vi "FindWedgeh.vi"(0 "Case Number":i32, 1 "cap theta":dbl[](array[numeric]) format="%.2f", 2 "rmin out":dbl format="%.2f", 3 "Sigma":dbl[](array[numeric]) format="%.2f", 4 "slice thetas":dbl[][](array[numeric]) format="%.4f", 5 "slice delay points in":i32, 6 "r values":T1 {"r5" format="%.2f"; "r4" format="%.2f"; "r3" format="%.2f"; "r2" format="%.2f"; "r1" format="%.2f"; "r0" format="%.2f"}, 7 "P constants":T3 {"Dtemp" format="%.2f"; "B" format="%.2f"; "A" format="%.2f"; "thetaw" format="%.2f"; "phih" format="%.2f"; "r" format="%.2f"}, 8 "strip":cluster{"Radius":dbl, "h":dbl, "a":dbl}={"Radius"=10.0, "h"=3.0, "a"=5.0} {"Radius" format="%.2f"; "a" format="%.2f"; "h" format="%.2f"}, 9 "P":cluster{"x":dbl, "y":dbl, "z":dbl}={"x"=1.0, "y"=-5.0, "z"=2.0} {"x" format="%.2f"; "z" format="%.2f"; "y" format="%.2f"}, 10 "Variables":T2={"sound spd (cm/s)"=150000, "time step (s)"=1e-09} {"time step (s)" format="%.2e"}, 11 "Transform matrix":dbl[][](array[numeric]) format="%.2f") -> (16 "h wedge":dbl[](graph), 18 "slice delay out":i32)   [LabVIEW 2022 SP3]
uses:
  <vilib>/Analysis/baseanly.llb/A x Vector.vi
  <vilib>/Analysis/NI_AALBase.lvlib
panel:
  out "x/y temp":T1 {"r5" format="%.2f"; "r4" format="%.2f"; "r3" format="%.2f"; "r2" format="%.2f"; "r1" format="%.2f"; "r0" format="%.2f"}
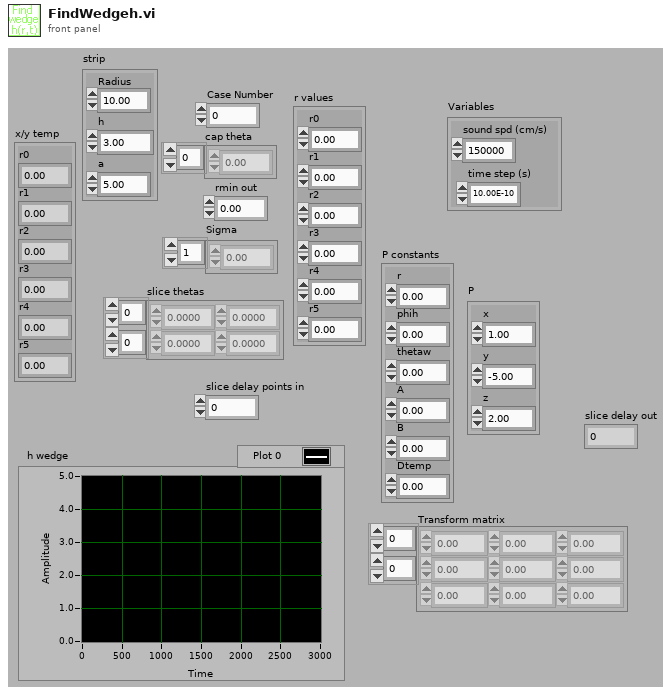
[diagram p1: front panel]
types:
  T1 = cluster{"r0":dbl, "r1":dbl, "r2":dbl, "r3":dbl, "r4":dbl, "r5":dbl}
  T2 = cluster{"sound spd (cm/s)":i32, "time step (s)":sgl}
  T3 = cluster{"r":dbl, "phih":dbl, "thetaw":dbl, "A":dbl, "B":dbl, "Dtemp":dbl}
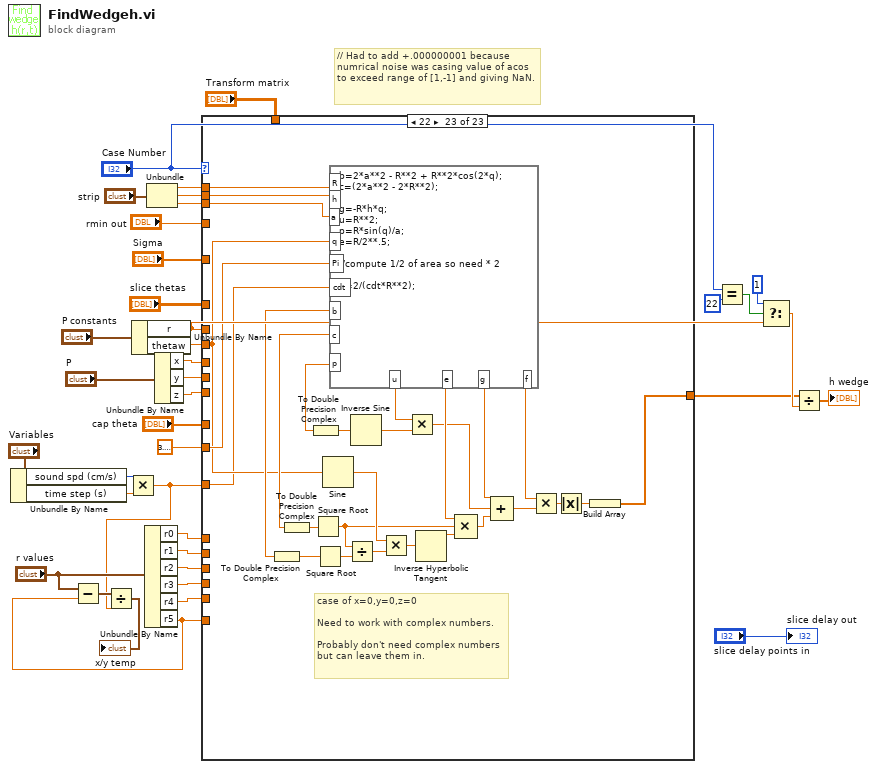
[diagram p0: block diagram]
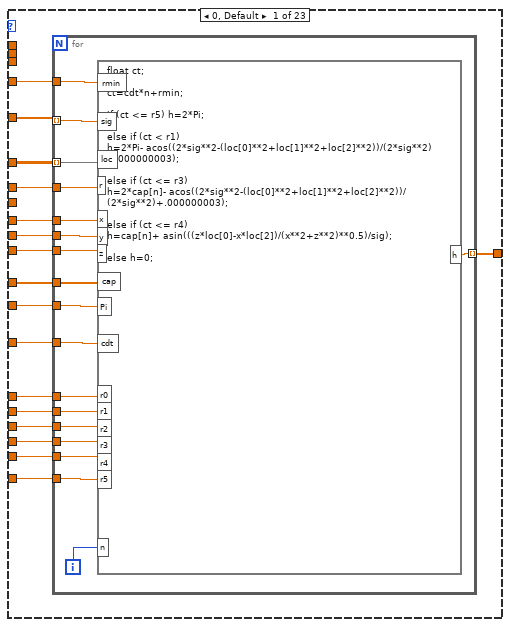
[diagram p2: hidden frame]
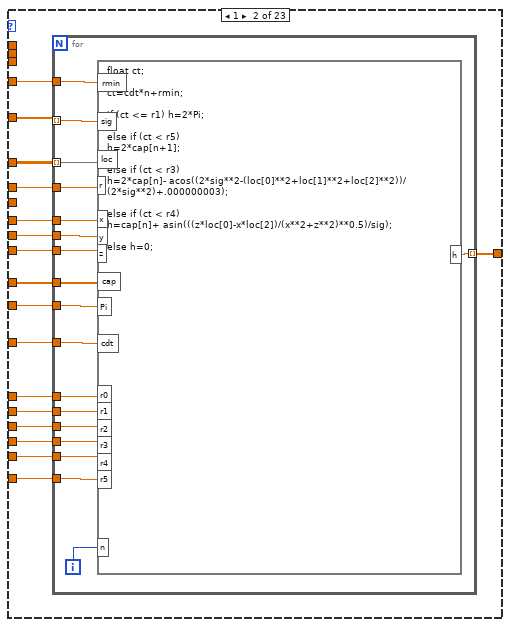
[diagram p3: hidden frame]
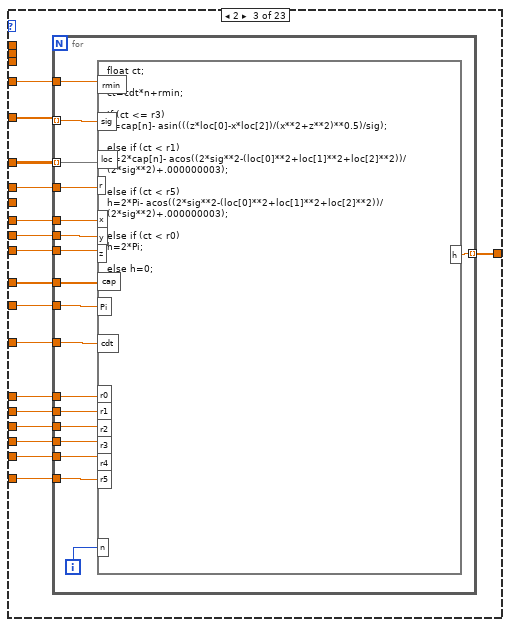
[diagram p4: hidden frame]
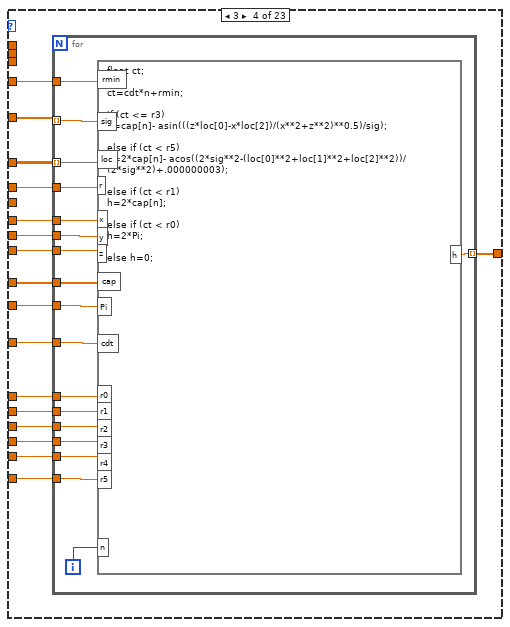
[diagram p5: hidden frame]
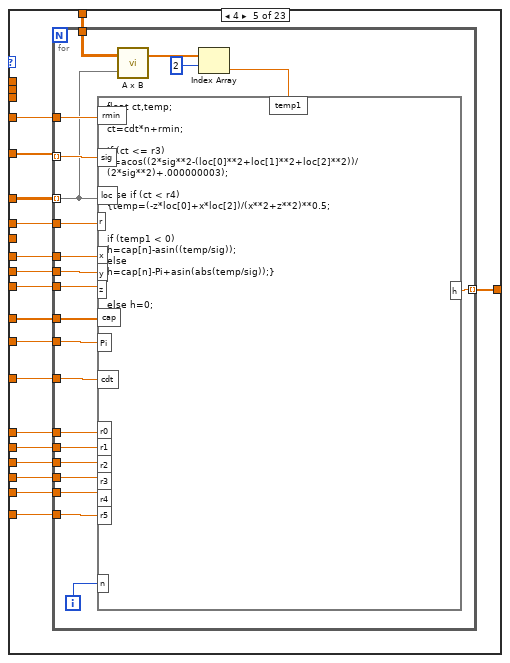
[diagram p6: hidden frame]
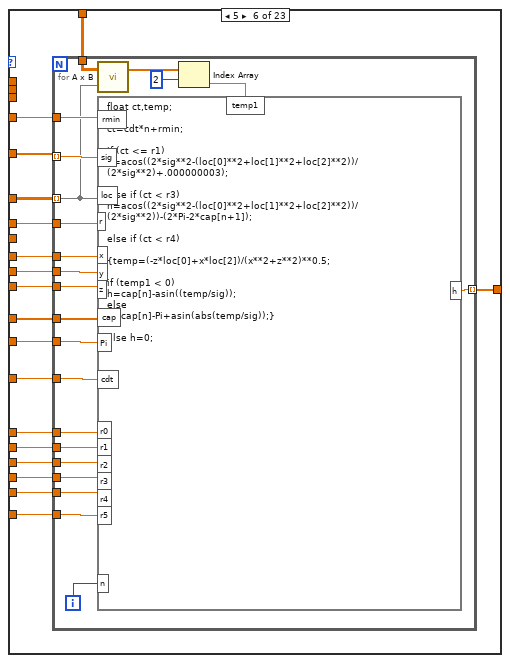
[diagram p7: hidden frame]
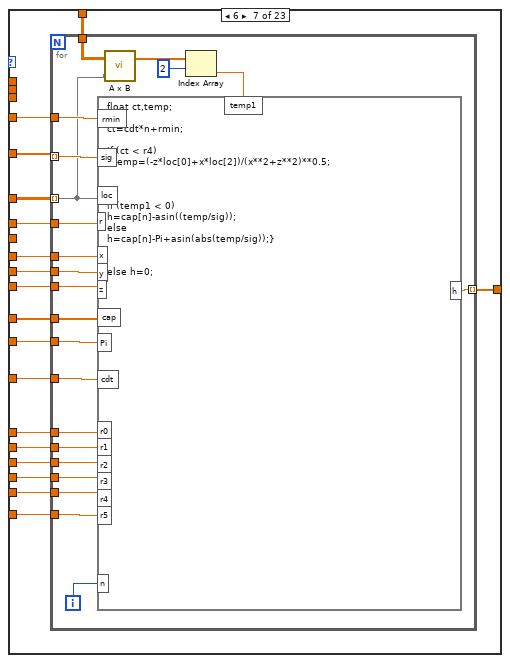
[diagram p8: hidden frame]
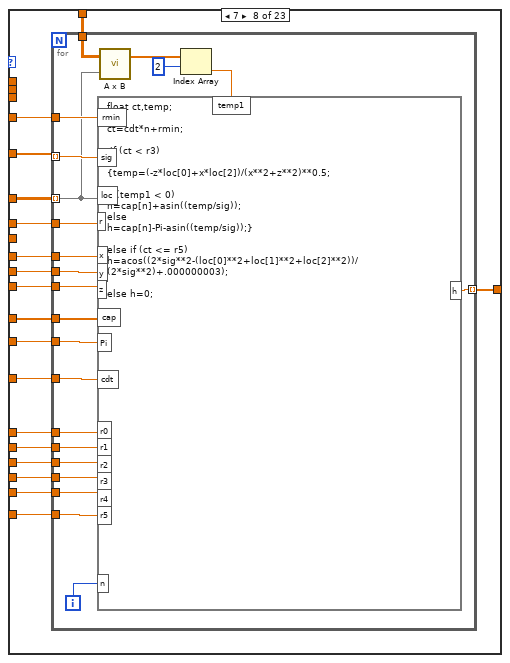
[diagram p9: hidden frame]
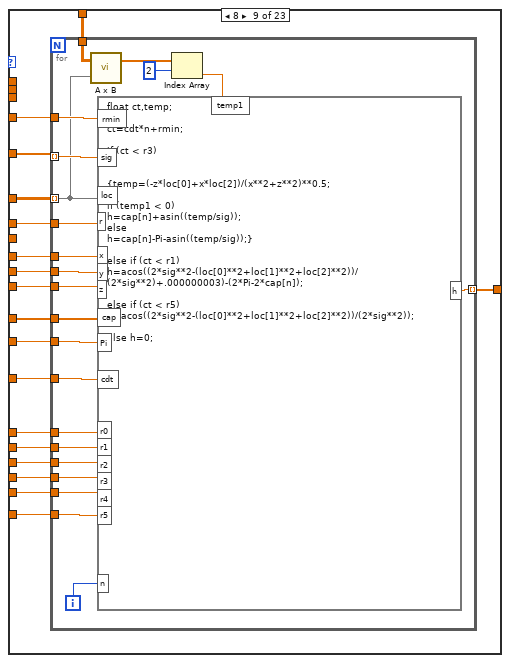
[diagram p10: hidden frame]
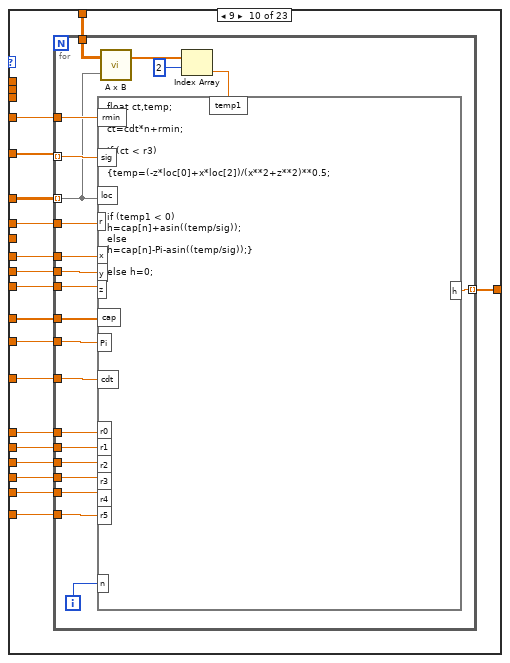
[diagram p11: hidden frame]
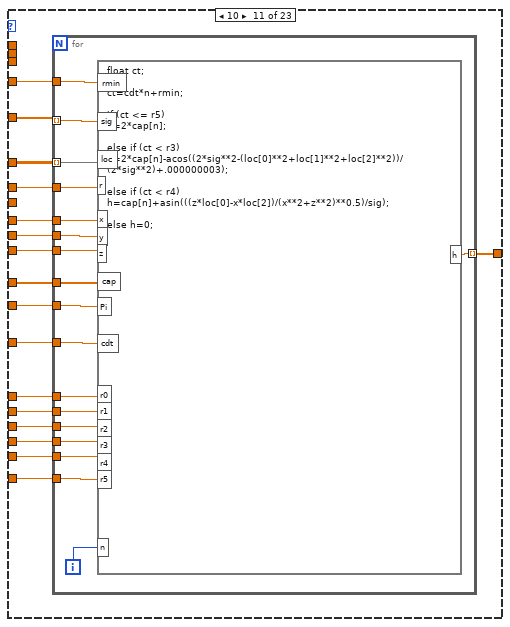
[diagram p12: hidden frame]
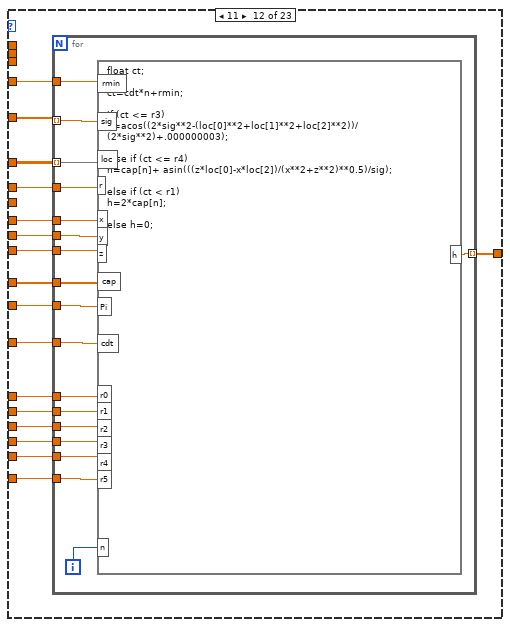
[diagram p13: hidden frame]
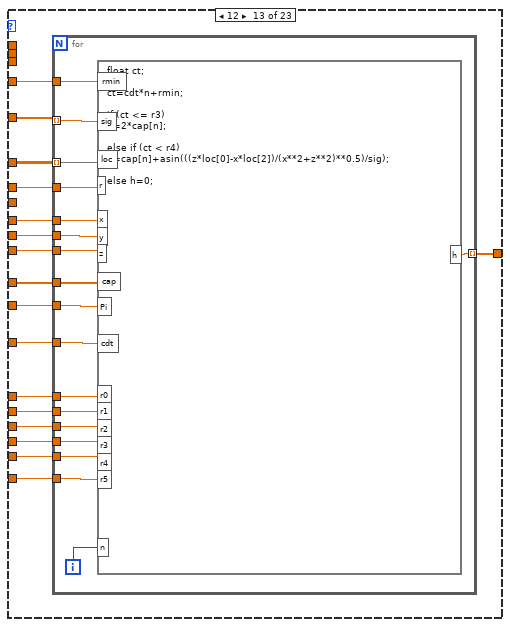
[diagram p14: hidden frame]
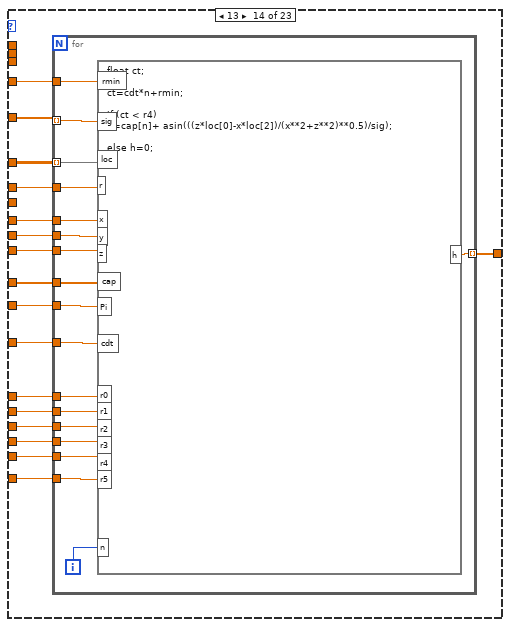
[diagram p15: hidden frame]
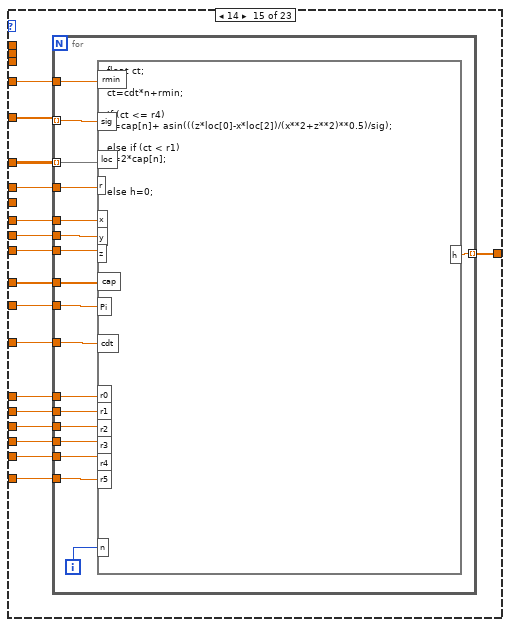
[diagram p16: hidden frame]
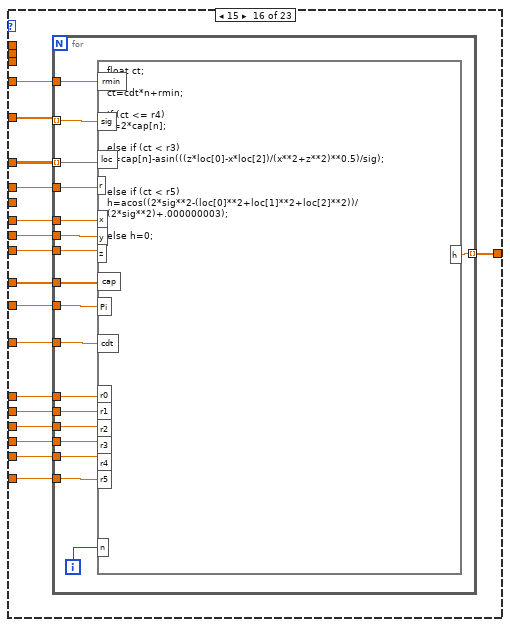
[diagram p17: hidden frame]
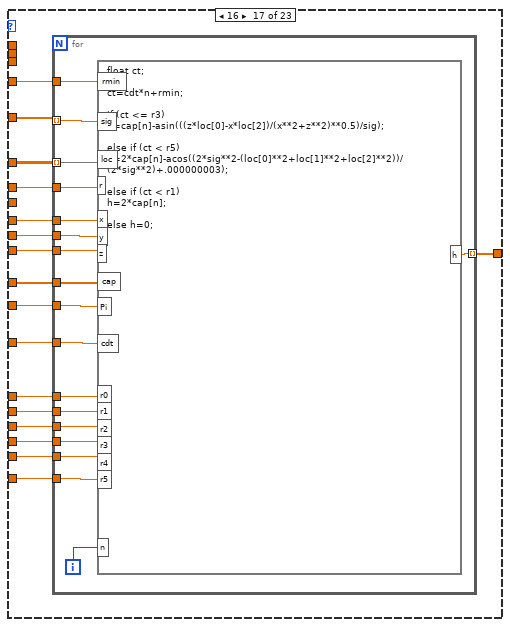
[diagram p18: hidden frame]
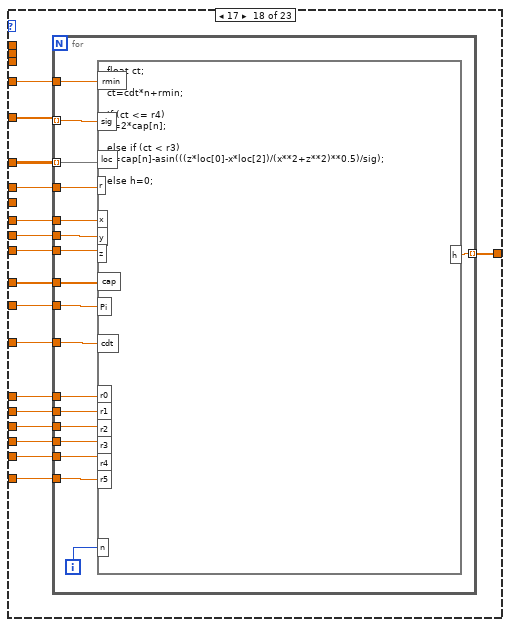
[diagram p19: hidden frame]
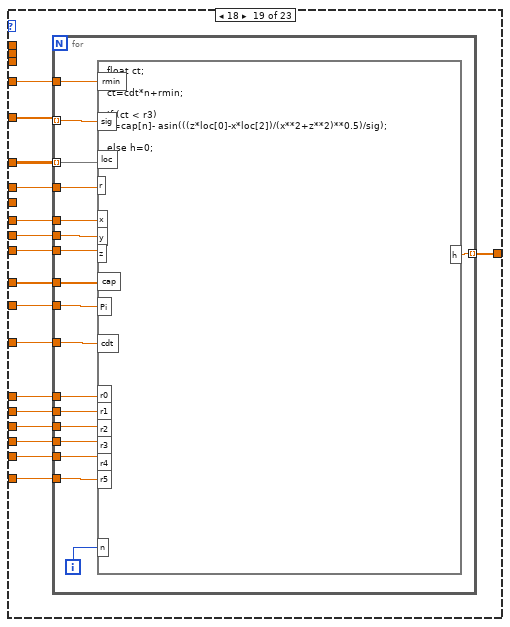
[diagram p20: hidden frame]
diagram:
  # "// Had to add +.000000001 because numrical noise was casing value of acos to exceed range of [1,-1] and giving NaN."
  n1 = Unbundle By Name("Variables") -> ("sound spd (cm/s)"=w26:i32, "time step (s)"=w7:sgl)
  n2 = Multiply(x=w26, y=w7) -> (x*y=w25:sgl)
  n3 = Unbundle By Name("P constants") -> ("r"=w8:dbl, "thetaw"=w18:dbl)
  n4 = Unbundle By Name("r values") -> ("r0"=w27:dbl, "r1"=w20:dbl, "r2"=w22:dbl, "r3"=w21:dbl, "r4"=w5:dbl, "r5"=w4:dbl)
  n5 = Subtract(x="r values", y=w4) -> (x-y=w30:T1)
  n6 = Divide(x=w30, y=w25) -> (x/y=→"x/y temp":T1)
  n7 = Unbundle("strip") -> ("Radius"=w10:dbl, "h"=w16:dbl, "a"=w15:dbl)
  n8 = Unbundle By Name("P") -> ("x"=w34:dbl, "y"=w33:dbl, "z"=w32:dbl)
  n9 = case shown="22" "Case Number" {
    tunnel: "cap theta" -> [w54 w89 w124 w159 w195 w235 w275 w315 w355 w395 w434 w469 w504 w539 w574 w609 w644 w679 w714 w749 w784 w819 _]
    tunnel: w25 -> [w55 w90 w125 w160 w196 w236 w276 w316 w356 w396 w435 w470 w505 w540 w575 w610 w645 w680 w715 w750 w785 w820 w846]
    tunnel: "slice thetas" -> [w41 w76 w111 w146 w182 w222 w262 w302 w342 w382 w421 w456 w491 w526 w561 w596 w631 w666 w701 w736 w771 w806 _]
    tunnel: w8 -> [w53 w88 w123 w158 w194 w234 w274 w314 w354 w394 w433 w468 w503 w538 w573 w608 w643 w678 w713 w748 w783 w818 _]
    tunnel: w27 -> [w52 w87 w122 w157 w193 w233 w273 w313 w353 w393 w432 w467 w502 w537 w572 w607 w642 w677 w712 w747 w782 w817 _]
    tunnel: w20 -> [w51 w86 w121 w156 w192 w232 w272 w312 w352 w392 w431 w466 w501 w536 w571 w606 w641 w676 w711 w746 w781 w816 _]
    tunnel: w22 -> [w50 w85 w120 w155 w191 w231 w271 w311 w351 w391 w430 w465 w500 w535 w570 w605 w640 w675 w710 w745 w780 w815 _]
    tunnel: w21 -> [w49 w84 w119 w154 w190 w230 w270 w310 w350 w390 w429 w464 w499 w534 w569 w604 w639 w674 w709 w744 w779 w814 _]
    tunnel: w5 -> [w48 w83 w118 w153 w189 w229 w269 w309 w349 w389 w428 w463 w498 w533 w568 w603 w638 w673 w708 w743 w778 w813 _]
    tunnel: w4 -> [w47 w82 w117 w152 w188 w228 w268 w308 w348 w388 w427 w462 w497 w532 w567 w602 w637 w672 w707 w742 w777 w812 _]
    tunnel: 3.141592653589793 -> [w46 w81 w116 w151 w187 w227 w267 w307 w347 w387 w426 w461 w496 w531 w566 w601 w636 w671 w706 w741 w776 w811 w866]
    tunnel: "Sigma" -> [w40 w75 w110 w145 w181 w221 w261 w301 w341 w381 w420 w455 w490 w525 w560 w595 w630 w665 w700 w735 w770 w805 _]
    tunnel: w34 -> [w45 w80 w115 w150 w186 w226 w266 w306 w346 w386 w425 w460 w495 w530 w565 w600 w635 w670 w705 w740 w775 w810 _]
    tunnel: w33 -> [w44 w79 w114 w149 w185 w225 w265 w305 w345 w385 w424 w459 w494 w529 w564 w599 w634 w669 w704 w739 w774 w809 _]
    tunnel: w32 -> [w43 w78 w113 w148 w184 w224 w264 w304 w344 w384 w423 w458 w493 w528 w563 w598 w633 w668 w703 w738 w773 w808 _]
    tunnel: [w42 w77 w112 w147 w183 w223 w263 w303 w343 w383 w422 w457 w492 w527 w562 w597 w632 w667 w702 w737 w772 w807 w867] -> w6
    tunnel: "rmin out" -> [w39 w74 w109 w144 w180 w220 w260 w300 w340 w380 w419 w454 w489 w524 w559 w594 w629 w664 w699 w734 w769 w804 _]
    tunnel: w18 -> [_ _ _ _ _ _ _ _ _ _ _ _ _ _ _ _ _ _ _ _ _ _ w857]
    tunnel: w10 -> [_ _ _ _ _ _ _ _ _ _ _ _ _ _ _ _ _ _ _ _ _ _ w865]
    tunnel: w16 -> [_ _ _ _ _ _ _ _ _ _ _ _ _ _ _ _ _ _ _ _ _ _ w864]
    tunnel: w15 -> [_ _ _ _ _ _ _ _ _ _ _ _ _ _ _ _ _ _ _ _ _ _ w863]
    tunnel: "Transform matrix" -> [_ _ _ _ w179 w219 w259 w299 w339 w379 _ _ _ _ _ _ _ _ _ _ _ _ _]
    frame 0, Default {
      n10 = for {
        tunnel: w55 -> [w67]
        tunnel: w41 -> [w57] mode=indexing
        tunnel: w54 -> [w59]
        tunnel: w53 -> [w61]
        tunnel: w52 -> [w73]
        tunnel: w51 -> [w72]
        tunnel: w50 -> [w71]
        tunnel: w49 -> [w70]
        tunnel: w48 -> [w69]
        tunnel: w47 -> [w68]
        tunnel: w46 -> [w65]
        tunnel: w45 -> [w64]
        tunnel: w44 -> [w63]
        tunnel: w43 -> [w62]
        tunnel: w40 -> [w60] mode=indexing
        tunnel: [w58] -> w42 mode=indexing
        tunnel: w39 -> [w56]
        i -> [w66]
        n11 = formula code="float ct;\n\nct=cdt*n+rmin;\n\nif (ct <= r5) h=2*Pi;\n\nelse if (ct < r1)\nh=2*Pi- acos((2*sig**2-(loc[0]**2+loc[1]**2+loc[2]**2))/(2*sig**2) +.000000003);\n\nelse if (ct <= r3)\nh=2*cap[n]- acos((2*sig**2-(loc[0]**2+loc[1]**2+loc[2]**2))/(2*sig**2)+.000000003);\n\nelse if (ct <= r4)\nh=cap[n]+ asin(((z*loc[0]-x*loc[2])/(x**2+z**2)**0.5)/sig);\n\nelse h=0;"("r0"=w73, "r1"=w72, "r2"=w71, "r3"=w70, "r4"=w69, "r5"=w68, "cdt"=w67, "n"=w66, "Pi"=w65, "x"=w64, "y"=w63, "z"=w62, "r"=w61, "sig"=w60, "loc"=w57, "cap"=w59, "rmin"=w56) -> ("h"=w58:dbl)
      }
    }
    frame 1 {
      n12 = for {
        tunnel: w90 -> [w102]
        tunnel: w76 -> [w92] mode=indexing
        tunnel: w89 -> [w94]
        tunnel: w88 -> [w96]
        tunnel: w87 -> [w108]
        tunnel: w86 -> [w107]
        tunnel: w85 -> [w106]
        tunnel: w84 -> [w105]
        tunnel: w83 -> [w104]
        tunnel: w82 -> [w103]
        tunnel: w81 -> [w100]
        tunnel: w80 -> [w99]
        tunnel: w79 -> [w98]
        tunnel: w78 -> [w97]
        tunnel: w75 -> [w95] mode=indexing
        tunnel: [w93] -> w77 mode=indexing
        tunnel: w74 -> [w91]
        i -> [w101]
        n13 = formula code="float ct;\n\nct=cdt*n+rmin;\n\nif (ct <= r1) h=2*Pi;\n\nelse if (ct < r5)\nh=2*cap[n+1];\n\nelse if (ct < r3)\nh=2*cap[n]- acos((2*sig**2-(loc[0]**2+loc[1]**2+loc[2]**2))/(2*sig**2)+.000000003);\n\nelse if (ct < r4)\nh=cap[n]+ asin(((z*loc[0]-x*loc[2])/(x**2+z**2)**0.5)/sig);\n\nelse h=0;"("r0"=w108, "r1"=w107, "r2"=w106, "r3"=w105, "r4"=w104, "r5"=w103, "cdt"=w102, "n"=w101, "Pi"=w100, "x"=w99, "y"=w98, "z"=w97, "r"=w96, "sig"=w95, "loc"=w92, "cap"=w94, "rmin"=w91) -> ("h"=w93:dbl)
      }
    }
    frame 2 {
      n14 = for {
        tunnel: w125 -> [w137]
        tunnel: w111 -> [w127] mode=indexing
        tunnel: w124 -> [w129]
        tunnel: w123 -> [w131]
        tunnel: w122 -> [w143]
        tunnel: w121 -> [w142]
        tunnel: w120 -> [w141]
        tunnel: w119 -> [w140]
        tunnel: w118 -> [w139]
        tunnel: w117 -> [w138]
        tunnel: w116 -> [w135]
        tunnel: w115 -> [w134]
        tunnel: w114 -> [w133]
        tunnel: w113 -> [w132]
        tunnel: w110 -> [w130] mode=indexing
        tunnel: [w128] -> w112 mode=indexing
        tunnel: w109 -> [w126]
        i -> [w136]
        n15 = formula code="float ct;\n\nct=cdt*n+rmin;\n\nif (ct <= r3)\nh=cap[n]- asin(((z*loc[0]-x*loc[2])/(x**2+z**2)**0.5)/sig);\n\nelse if (ct < r1)\nh=2*cap[n]- acos((2*sig**2-(loc[0]**2+loc[1]**2+loc[2]**2))/(2*sig**2)+.000000003);\n\nelse if (ct < r5)\nh=2*Pi- acos((2*sig**2-(loc[0]**2+loc[1]**2+loc[2]**2))/(2*sig**2)+.000000003);\n\nelse if (ct < r0)\nh=2*Pi;\n\nelse h=0;"("r0"=w143, "r1"=w142, "r2"=w141, "r3"=w140, "r4"=w139, "r5"=w138, "cdt"=w137, "n"=w136, "Pi"=w135, "x"=w134, "y"=w133, "z"=w132, "r"=w131, "sig"=w130, "loc"=w127, "cap"=w129, "rmin"=w126) -> ("h"=w128:dbl)
      }
    }
    frame 3 {
      n16 = for {
        tunnel: w160 -> [w172]
        tunnel: w146 -> [w162] mode=indexing
        tunnel: w159 -> [w164]
        tunnel: w158 -> [w166]
        tunnel: w157 -> [w178]
        tunnel: w156 -> [w177]
        tunnel: w155 -> [w176]
        tunnel: w154 -> [w175]
        tunnel: w153 -> [w174]
        tunnel: w152 -> [w173]
        tunnel: w151 -> [w170]
        tunnel: w150 -> [w169]
        tunnel: w149 -> [w168]
        tunnel: w148 -> [w167]
        tunnel: w145 -> [w165] mode=indexing
        tunnel: [w163] -> w147 mode=indexing
        tunnel: w144 -> [w161]
        i -> [w171]
        n17 = formula code="float ct;\n\nct=cdt*n+rmin;\n\nif (ct <= r3)\nh=cap[n]- asin(((z*loc[0]-x*loc[2])/(x**2+z**2)**0.5)/sig);\n\nelse if (ct < r5)\nh=2*cap[n]- acos((2*sig**2-(loc[0]**2+loc[1]**2+loc[2]**2))/(2*sig**2)+.000000003);\n\nelse if (ct < r1)\nh=2*cap[n];\n\nelse if (ct < r0)\nh=2*Pi;\n\nelse h=0;"("r0"=w178, "r1"=w177, "r2"=w176, "r3"=w175, "r4"=w174, "r5"=w173, "cdt"=w172, "n"=w171, "Pi"=w170, "x"=w169, "y"=w168, "z"=w167, "r"=w166, "sig"=w165, "loc"=w162, "cap"=w164, "rmin"=w161) -> ("h"=w163:dbl)
      }
    }
    frame 4 {
      n18 = for {
        tunnel: w196 -> [w212]
        tunnel: w182 -> [w198] mode=indexing
        tunnel: w195 -> [w204]
        tunnel: w194 -> [w206]
        tunnel: w193 -> [w218]
        tunnel: w192 -> [w217]
        tunnel: w191 -> [w216]
        tunnel: w190 -> [w215]
        tunnel: w189 -> [w214]
        tunnel: w188 -> [w213]
        tunnel: w187 -> [w210]
        tunnel: w186 -> [w209]
        tunnel: w185 -> [w208]
        tunnel: w184 -> [w207]
        tunnel: w181 -> [w205] mode=indexing
        tunnel: [w203] -> w183 mode=indexing
        tunnel: w180 -> [w202]
        tunnel: w179 -> [w199]
        i -> [w211]
        n19 = call-poly <vilib>:"A x B.vi"("Vector"=w198, "A"=w199) -> ("A x Vector"=w200:dbl[])  [unwired: 1 out]
        n20 = Index Array(array=w200, index=2) -> (element=w197:dbl)
        n21 = formula code="float ct,temp;\n\nct=cdt*n+rmin;\n\nif (ct <= r3)\nh=acos((2*sig**2-(loc[0]**2+loc[1]**2+loc[2]**2))/(2*sig**2)+.000000003);\n\nelse if (ct < r4)\n{temp=(-z*loc[0]+x*loc[2])/(x**2+z**2)**0.5;\n\n\nif (temp1 < 0)\nh=cap[n]-asin((temp/sig));\nelse \nh=cap[n]-Pi+asin(abs(temp/sig));}\n\n\nelse h=0;"("r0"=w218, "r1"=w217, "r2"=w216, "r3"=w215, "r4"=w214, "r5"=w213, "cdt"=w212, "n"=w211, "Pi"=w210, "x"=w209, "y"=w208, "z"=w207, "r"=w206, "sig"=w205, "loc"=w198, "cap"=w204, "rmin"=w202, "temp1"=w197) -> ("h"=w203:dbl)
      }
    }
    frame 5 {
      n22 = for {
        tunnel: w236 -> [w252]
        tunnel: w222 -> [w239] mode=indexing
        tunnel: w235 -> [w240]
        tunnel: w234 -> [w246]
        tunnel: w233 -> [w258]
        tunnel: w232 -> [w257]
        tunnel: w231 -> [w256]
        tunnel: w230 -> [w255]
        tunnel: w229 -> [w254]
        tunnel: w228 -> [w253]
        tunnel: w227 -> [w250]
        tunnel: w226 -> [w249]
        tunnel: w225 -> [w248]
        tunnel: w224 -> [w247]
        tunnel: w221 -> [w245] mode=indexing
        tunnel: [w244] -> w223 mode=indexing
        tunnel: w220 -> [w243]
        tunnel: w219 -> [w237]
        i -> [w251]
        n23 = call-poly <vilib>:"A x B.vi"("Vector"=w239, "A"=w237) -> ("A x Vector"=w238:dbl[])  [unwired: 1 out]
        n24 = Index Array(array=w238, index=2) -> (element=w241:dbl)
        n25 = formula code="float ct,temp;\n\nct=cdt*n+rmin;\n\nif (ct <= r1)\nh=acos((2*sig**2-(loc[0]**2+loc[1]**2+loc[2]**2))/(2*sig**2)+.000000003);\n\nelse if (ct < r3)\nh=acos((2*sig**2-(loc[0]**2+loc[1]**2+loc[2]**2))/(2*sig**2))-(2*Pi-2*cap[n+1]);\n\nelse if (ct < r4)\n\n{temp=(-z*loc[0]+x*loc[2])/(x**2+z**2)**0.5;\n\nif (temp1 < 0)\nh=cap[n]-asin((temp/sig));\nelse \nh=cap[n]-Pi+asin(abs(temp/sig));}\n\nelse h=0;"("r0"=w258, "r1"=w257, "r2"=w256, "r3"=w255, "r4"=w254, "r5"=w253, "cdt"=w252, "n"=w251, "Pi"=w250, "x"=w249, "y"=w248, "z"=w247, "r"=w246, "sig"=w245, "loc"=w239, "cap"=w240, "rmin"=w243, "temp1"=w241) -> ("h"=w244:dbl)
      }
    }
    frame 6 {
      n26 = for {
        tunnel: w276 -> [w292]
        tunnel: w262 -> [w278] mode=indexing
        tunnel: w275 -> [w284]
        tunnel: w274 -> [w286]
        tunnel: w273 -> [w298]
        tunnel: w272 -> [w297]
        tunnel: w271 -> [w296]
        tunnel: w270 -> [w295]
        tunnel: w269 -> [w294]
        tunnel: w268 -> [w293]
        tunnel: w267 -> [w290]
        tunnel: w266 -> [w289]
        tunnel: w265 -> [w288]
        tunnel: w264 -> [w287]
        tunnel: w261 -> [w285] mode=indexing
        tunnel: [w283] -> w263 mode=indexing
        tunnel: w260 -> [w282]
        tunnel: w259 -> [w279]
        i -> [w291]
        n27 = call-poly <vilib>:"A x B.vi"("Vector"=w278, "A"=w279) -> ("A x Vector"=w280:dbl[])  [unwired: 1 out]
        n28 = Index Array(array=w280, index=2) -> (element=w277:dbl)
        n29 = formula code="float ct,temp;\n\nct=cdt*n+rmin;\n\nif (ct < r4)\n{temp=(-z*loc[0]+x*loc[2])/(x**2+z**2)**0.5;\n\n\n\nif (temp1 < 0)\nh=cap[n]-asin((temp/sig));\nelse \nh=cap[n]-Pi+asin(abs(temp/sig));}\n\n\nelse h=0;"("r0"=w298, "r1"=w297, "r2"=w296, "r3"=w295, "r4"=w294, "r5"=w293, "cdt"=w292, "n"=w291, "Pi"=w290, "x"=w289, "y"=w288, "z"=w287, "r"=w286, "sig"=w285, "loc"=w278, "cap"=w284, "rmin"=w282, "temp1"=w277) -> ("h"=w283:dbl)
      }
    }
    frame 7 {
      n30 = for {
        tunnel: w316 -> [w332]
        tunnel: w302 -> [w318] mode=indexing
        tunnel: w315 -> [w324]
        tunnel: w314 -> [w326]
        tunnel: w313 -> [w338]
        tunnel: w312 -> [w337]
        tunnel: w311 -> [w336]
        tunnel: w310 -> [w335]
        tunnel: w309 -> [w334]
        tunnel: w308 -> [w333]
        tunnel: w307 -> [w330]
        tunnel: w306 -> [w329]
        tunnel: w305 -> [w328]
        tunnel: w304 -> [w327]
        tunnel: w301 -> [w325] mode=indexing
        tunnel: [w323] -> w303 mode=indexing
        tunnel: w300 -> [w322]
        tunnel: w299 -> [w319]
        i -> [w331]
        n31 = call-poly <vilib>:"A x B.vi"("Vector"=w318, "A"=w319) -> ("A x Vector"=w320:dbl[])  [unwired: 1 out]
        n32 = Index Array(array=w320, index=2) -> (element=w317:dbl)
        n33 = formula code="float ct,temp;\n\nct=cdt*n+rmin;\n\n if (ct < r3)\n\n{temp=(-z*loc[0]+x*loc[2])/(x**2+z**2)**0.5;\n\nif (temp1 < 0)\nh=cap[n]+asin((temp/sig));\nelse \nh=cap[n]-Pi-asin((temp/sig));}\n\nelse if (ct <= r5)\nh=acos((2*sig**2-(loc[0]**2+loc[1]**2+loc[2]**2))/(2*sig**2)+.000000003);\n\nelse h=0;"("r0"=w338, "r1"=w337, "r2"=w336, "r3"=w335, "r4"=w334, "r5"=w333, "cdt"=w332, "n"=w331, "Pi"=w330, "x"=w329, "y"=w328, "z"=w327, "r"=w326, "sig"=w325, "loc"=w318, "cap"=w324, "rmin"=w322, "temp1"=w317) -> ("h"=w323:dbl)
      }
    }
    frame 8 {
      n34 = for {
        tunnel: w356 -> [w372]
        tunnel: w342 -> [w358] mode=indexing
        tunnel: w355 -> [w364]
        tunnel: w354 -> [w366]
        tunnel: w353 -> [w378]
        tunnel: w352 -> [w377]
        tunnel: w351 -> [w376]
        tunnel: w350 -> [w375]
        tunnel: w349 -> [w374]
        tunnel: w348 -> [w373]
        tunnel: w347 -> [w370]
        tunnel: w346 -> [w369]
        tunnel: w345 -> [w368]
        tunnel: w344 -> [w367]
        tunnel: w341 -> [w365] mode=indexing
        tunnel: [w363] -> w343 mode=indexing
        tunnel: w340 -> [w362]
        tunnel: w339 -> [w359]
        i -> [w371]
        n35 = call-poly <vilib>:"A x B.vi"("Vector"=w358, "A"=w359) -> ("A x Vector"=w360:dbl[])  [unwired: 1 out]
        n36 = Index Array(array=w360, index=2) -> (element=w357:dbl)
        n37 = formula code="float ct,temp;\n\nct=cdt*n+rmin;\n\nif (ct < r3)\n\n\n{temp=(-z*loc[0]+x*loc[2])/(x**2+z**2)**0.5;\n\nif (temp1 < 0)\nh=cap[n]+asin((temp/sig));\nelse \nh=cap[n]-Pi-asin((temp/sig));}\n\nelse if (ct < r1)\nh=acos((2*sig**2-(loc[0]**2+loc[1]**2+loc[2]**2))/(2*sig**2)+.000000003)-(2*Pi-2*cap[n]);\n\nelse if (ct < r5)\nh=acos((2*sig**2-(loc[0]**2+loc[1]**2+loc[2]**2))/(2*sig**2));\n\nelse h=0;"("r0"=w378, "r1"=w377, "r2"=w376, "r3"=w375, "r4"=w374, "r5"=w373, "cdt"=w372, "n"=w371, "Pi"=w370, "x"=w369, "y"=w368, "z"=w367, "r"=w366, "sig"=w365, "loc"=w358, "cap"=w364, "rmin"=w362, "temp1"=w357) -> ("h"=w363:dbl)
      }
    }
    frame 9 {
      n38 = for {
        tunnel: w396 -> [w412]
        tunnel: w382 -> [w398] mode=indexing
        tunnel: w395 -> [w404]
        tunnel: w394 -> [w406]
        tunnel: w393 -> [w418]
        tunnel: w392 -> [w417]
        tunnel: w391 -> [w416]
        tunnel: w390 -> [w415]
        tunnel: w389 -> [w414]
        tunnel: w388 -> [w413]
        tunnel: w387 -> [w410]
        tunnel: w386 -> [w409]
        tunnel: w385 -> [w408]
        tunnel: w384 -> [w407]
        tunnel: w381 -> [w405] mode=indexing
        tunnel: [w403] -> w383 mode=indexing
        tunnel: w380 -> [w402]
        tunnel: w379 -> [w399]
        i -> [w411]
        n39 = call-poly <vilib>:"A x B.vi"("Vector"=w398, "A"=w399) -> ("A x Vector"=w400:dbl[])  [unwired: 1 out]
        n40 = Index Array(array=w400, index=2) -> (element=w397:dbl)
        n41 = formula code="float ct,temp;\n\nct=cdt*n+rmin;\n\nif (ct < r3)\n\n{temp=(-z*loc[0]+x*loc[2])/(x**2+z**2)**0.5;\n\n\n\nif (temp1 < 0)\nh=cap[n]+asin((temp/sig));\nelse \nh=cap[n]-Pi-asin((temp/sig));}\n\nelse h=0;"("r0"=w418, "r1"=w417, "r2"=w416, "r3"=w415, "r4"=w414, "r5"=w413, "cdt"=w412, "n"=w411, "Pi"=w410, "x"=w409, "y"=w408, "z"=w407, "r"=w406, "sig"=w405, "loc"=w398, "cap"=w404, "rmin"=w402, "temp1"=w397) -> ("h"=w403:dbl)
      }
    }
    frame 10 {
      n42 = for {
        tunnel: w435 -> [w447]
        tunnel: w421 -> [w437] mode=indexing
        tunnel: w434 -> [w439]
        tunnel: w433 -> [w441]
        tunnel: w432 -> [w453]
        tunnel: w431 -> [w452]
        tunnel: w430 -> [w451]
        tunnel: w429 -> [w450]
        tunnel: w428 -> [w449]
        tunnel: w427 -> [w448]
        tunnel: w426 -> [w445]
        tunnel: w425 -> [w444]
        tunnel: w424 -> [w443]
        tunnel: w423 -> [w442]
        tunnel: w420 -> [w440] mode=indexing
        tunnel: [w438] -> w422 mode=indexing
        tunnel: w419 -> [w436]
        i -> [w446]
        n43 = formula code="float ct;\n\nct=cdt*n+rmin;\n\nif (ct <= r5)\nh=2*cap[n];\n\nelse if (ct < r3)\nh=2*cap[n]-acos((2*sig**2-(loc[0]**2+loc[1]**2+loc[2]**2))/(2*sig**2)+.000000003);\n\nelse if (ct < r4)\nh=cap[n]+asin(((z*loc[0]-x*loc[2])/(x**2+z**2)**0.5)/sig);\n\nelse h=0;"("r0"=w453, "r1"=w452, "r2"=w451, "r3"=w450, "r4"=w449, "r5"=w448, "cdt"=w447, "n"=w446, "Pi"=w445, "x"=w444, "y"=w443, "z"=w442, "r"=w441, "sig"=w440, "loc"=w437, "cap"=w439, "rmin"=w436) -> ("h"=w438:dbl)
      }
    }
    frame 11 {
      n44 = for {
        tunnel: w470 -> [w482]
        tunnel: w456 -> [w472] mode=indexing
        tunnel: w469 -> [w474]
        tunnel: w468 -> [w476]
        tunnel: w467 -> [w488]
        tunnel: w466 -> [w487]
        tunnel: w465 -> [w486]
        tunnel: w464 -> [w485]
        tunnel: w463 -> [w484]
        tunnel: w462 -> [w483]
        tunnel: w461 -> [w480]
        tunnel: w460 -> [w479]
        tunnel: w459 -> [w478]
        tunnel: w458 -> [w477]
        tunnel: w455 -> [w475] mode=indexing
        tunnel: [w473] -> w457 mode=indexing
        tunnel: w454 -> [w471]
        i -> [w481]
        n45 = formula code="float ct;\n\nct=cdt*n+rmin;\n\nif (ct <= r3)\nh=acos((2*sig**2-(loc[0]**2+loc[1]**2+loc[2]**2))/(2*sig**2)+.000000003);\n\nelse if (ct <= r4)\nh=cap[n]+ asin(((z*loc[0]-x*loc[2])/(x**2+z**2)**0.5)/sig);\n\nelse if (ct < r1)\nh=2*cap[n];\n\nelse h=0;"("r0"=w488, "r1"=w487, "r2"=w486, "r3"=w485, "r4"=w484, "r5"=w483, "cdt"=w482, "n"=w481, "Pi"=w480, "x"=w479, "y"=w478, "z"=w477, "r"=w476, "sig"=w475, "loc"=w472, "cap"=w474, "rmin"=w471) -> ("h"=w473:dbl)
      }
    }
    frame 12 {
      n46 = for {
        tunnel: w505 -> [w517]
        tunnel: w491 -> [w507] mode=indexing
        tunnel: w504 -> [w509]
        tunnel: w503 -> [w511]
        tunnel: w502 -> [w523]
        tunnel: w501 -> [w522]
        tunnel: w500 -> [w521]
        tunnel: w499 -> [w520]
        tunnel: w498 -> [w519]
        tunnel: w497 -> [w518]
        tunnel: w496 -> [w515]
        tunnel: w495 -> [w514]
        tunnel: w494 -> [w513]
        tunnel: w493 -> [w512]
        tunnel: w490 -> [w510] mode=indexing
        tunnel: [w508] -> w492 mode=indexing
        tunnel: w489 -> [w506]
        i -> [w516]
        n47 = formula code="float ct;\n\nct=cdt*n+rmin;\n\nif (ct <= r3)\nh=2*cap[n];\n\nelse if (ct < r4)\nh=cap[n]+asin(((z*loc[0]-x*loc[2])/(x**2+z**2)**0.5)/sig);\n\nelse h=0;"("r0"=w523, "r1"=w522, "r2"=w521, "r3"=w520, "r4"=w519, "r5"=w518, "cdt"=w517, "n"=w516, "Pi"=w515, "x"=w514, "y"=w513, "z"=w512, "r"=w511, "sig"=w510, "loc"=w507, "cap"=w509, "rmin"=w506) -> ("h"=w508:dbl)
      }
    }
    frame 13 {
      n48 = for {
        tunnel: w540 -> [w552]
        tunnel: w526 -> [w542] mode=indexing
        tunnel: w539 -> [w544]
        tunnel: w538 -> [w546]
        tunnel: w537 -> [w558]
        tunnel: w536 -> [w557]
        tunnel: w535 -> [w556]
        tunnel: w534 -> [w555]
        tunnel: w533 -> [w554]
        tunnel: w532 -> [w553]
        tunnel: w531 -> [w550]
        tunnel: w530 -> [w549]
        tunnel: w529 -> [w548]
        tunnel: w528 -> [w547]
        tunnel: w525 -> [w545] mode=indexing
        tunnel: [w543] -> w527 mode=indexing
        tunnel: w524 -> [w541]
        i -> [w551]
        n49 = formula code="float ct;\n\nct=cdt*n+rmin;\n\nif (ct < r4)\nh=cap[n]+ asin(((z*loc[0]-x*loc[2])/(x**2+z**2)**0.5)/sig);\n\nelse h=0;"("r0"=w558, "r1"=w557, "r2"=w556, "r3"=w555, "r4"=w554, "r5"=w553, "cdt"=w552, "n"=w551, "Pi"=w550, "x"=w549, "y"=w548, "z"=w547, "r"=w546, "sig"=w545, "loc"=w542, "cap"=w544, "rmin"=w541) -> ("h"=w543:dbl)
      }
    }
    frame 14 {
      n50 = for {
        tunnel: w575 -> [w587]
        tunnel: w561 -> [w577] mode=indexing
        tunnel: w574 -> [w579]
        tunnel: w573 -> [w581]
        tunnel: w572 -> [w593]
        tunnel: w571 -> [w592]
        tunnel: w570 -> [w591]
        tunnel: w569 -> [w590]
        tunnel: w568 -> [w589]
        tunnel: w567 -> [w588]
        tunnel: w566 -> [w585]
        tunnel: w565 -> [w584]
        tunnel: w564 -> [w583]
        tunnel: w563 -> [w582]
        tunnel: w560 -> [w580] mode=indexing
        tunnel: [w578] -> w562 mode=indexing
        tunnel: w559 -> [w576]
        i -> [w586]
        n51 = formula code="float ct;\n\nct=cdt*n+rmin;\n\nif (ct <= r4)\nh=cap[n]+ asin(((z*loc[0]-x*loc[2])/(x**2+z**2)**0.5)/sig);\n\nelse if (ct < r1)\nh=2*cap[n];\n\n\nelse h=0;"("r0"=w593, "r1"=w592, "r2"=w591, "r3"=w590, "r4"=w589, "r5"=w588, "cdt"=w587, "n"=w586, "Pi"=w585, "x"=w584, "y"=w583, "z"=w582, "r"=w581, "sig"=w580, "loc"=w577, "cap"=w579, "rmin"=w576) -> ("h"=w578:dbl)
      }
    }
    frame 15 {
      n52 = for {
        tunnel: w610 -> [w622]
        tunnel: w596 -> [w612] mode=indexing
        tunnel: w609 -> [w614]
        tunnel: w608 -> [w616]
        tunnel: w607 -> [w628]
        tunnel: w606 -> [w627]
        tunnel: w605 -> [w626]
        tunnel: w604 -> [w625]
        tunnel: w603 -> [w624]
        tunnel: w602 -> [w623]
        tunnel: w601 -> [w620]
        tunnel: w600 -> [w619]
        tunnel: w599 -> [w618]
        tunnel: w598 -> [w617]
        tunnel: w595 -> [w615] mode=indexing
        tunnel: [w613] -> w597 mode=indexing
        tunnel: w594 -> [w611]
        i -> [w621]
        n53 = formula code="float ct;\n\nct=cdt*n+rmin;\n\nif (ct <= r4)\nh=2*cap[n];\n\nelse if (ct < r3)\nh=cap[n]-asin(((z*loc[0]-x*loc[2])/(x**2+z**2)**0.5)/sig);\n\n\nelse if (ct < r5)\nh=acos((2*sig**2-(loc[0]**2+loc[1]**2+loc[2]**2))/(2*sig**2)+.000000003);\n\nelse h=0;"("r0"=w628, "r1"=w627, "r2"=w626, "r3"=w625, "r4"=w624, "r5"=w623, "cdt"=w622, "n"=w621, "Pi"=w620, "x"=w619, "y"=w618, "z"=w617, "r"=w616, "sig"=w615, "loc"=w612, "cap"=w614, "rmin"=w611) -> ("h"=w613:dbl)
      }
    }
    frame 16 {
      n54 = for {
        tunnel: w645 -> [w657]
        tunnel: w631 -> [w647] mode=indexing
        tunnel: w644 -> [w649]
        tunnel: w643 -> [w651]
        tunnel: w642 -> [w663]
        tunnel: w641 -> [w662]
        tunnel: w640 -> [w661]
        tunnel: w639 -> [w660]
        tunnel: w638 -> [w659]
        tunnel: w637 -> [w658]
        tunnel: w636 -> [w655]
        tunnel: w635 -> [w654]
        tunnel: w634 -> [w653]
        tunnel: w633 -> [w652]
        tunnel: w630 -> [w650] mode=indexing
        tunnel: [w648] -> w632 mode=indexing
        tunnel: w629 -> [w646]
        i -> [w656]
        n55 = formula code="float ct;\n\nct=cdt*n+rmin;\n\nif (ct <= r3)\nh=cap[n]-asin(((z*loc[0]-x*loc[2])/(x**2+z**2)**0.5)/sig);\n\nelse if (ct < r5)\nh=2*cap[n]-acos((2*sig**2-(loc[0]**2+loc[1]**2+loc[2]**2))/(2*sig**2)+.000000003);\n\nelse if (ct < r1)\nh=2*cap[n];\n\nelse h=0;"("r0"=w663, "r1"=w662, "r2"=w661, "r3"=w660, "r4"=w659, "r5"=w658, "cdt"=w657, "n"=w656, "Pi"=w655, "x"=w654, "y"=w653, "z"=w652, "r"=w651, "sig"=w650, "loc"=w647, "cap"=w649, "rmin"=w646) -> ("h"=w648:dbl)
      }
    }
    frame 17 {
      n56 = for {
        tunnel: w680 -> [w692]
        tunnel: w666 -> [w682] mode=indexing
        tunnel: w679 -> [w684]
        tunnel: w678 -> [w686]
        tunnel: w677 -> [w698]
        tunnel: w676 -> [w697]
        tunnel: w675 -> [w696]
        tunnel: w674 -> [w695]
        tunnel: w673 -> [w694]
        tunnel: w672 -> [w693]
        tunnel: w671 -> [w690]
        tunnel: w670 -> [w689]
        tunnel: w669 -> [w688]
        tunnel: w668 -> [w687]
        tunnel: w665 -> [w685] mode=indexing
        tunnel: [w683] -> w667 mode=indexing
        tunnel: w664 -> [w681]
        i -> [w691]
        n57 = formula code="float ct;\n\nct=cdt*n+rmin;\n\nif (ct <= r4)\nh=2*cap[n];\n\nelse if (ct < r3)\nh=cap[n]-asin(((z*loc[0]-x*loc[2])/(x**2+z**2)**0.5)/sig);\n\nelse h=0;"("r0"=w698, "r1"=w697, "r2"=w696, "r3"=w695, "r4"=w694, "r5"=w693, "cdt"=w692, "n"=w691, "Pi"=w690, "x"=w689, "y"=w688, "z"=w687, "r"=w686, "sig"=w685, "loc"=w682, "cap"=w684, "rmin"=w681) -> ("h"=w683:dbl)
      }
    }
    frame 18 {
      n58 = for {
        tunnel: w715 -> [w727]
        tunnel: w701 -> [w717] mode=indexing
        tunnel: w714 -> [w719]
        tunnel: w713 -> [w721]
        tunnel: w712 -> [w733]
        tunnel: w711 -> [w732]
        tunnel: w710 -> [w731]
        tunnel: w709 -> [w730]
        tunnel: w708 -> [w729]
        tunnel: w707 -> [w728]
        tunnel: w706 -> [w725]
        tunnel: w705 -> [w724]
        tunnel: w704 -> [w723]
        tunnel: w703 -> [w722]
        tunnel: w700 -> [w720] mode=indexing
        tunnel: [w718] -> w702 mode=indexing
        tunnel: w699 -> [w716]
        i -> [w726]
        n59 = formula code="float ct;\n\nct=cdt*n+rmin;\n\nif (ct < r3)\nh=cap[n]- asin(((z*loc[0]-x*loc[2])/(x**2+z**2)**0.5)/sig);\n\nelse h=0;"("r0"=w733, "r1"=w732, "r2"=w731, "r3"=w730, "r4"=w729, "r5"=w728, "cdt"=w727, "n"=w726, "Pi"=w725, "x"=w724, "y"=w723, "z"=w722, "r"=w721, "sig"=w720, "loc"=w717, "cap"=w719, "rmin"=w716) -> ("h"=w718:dbl)
      }
    }
    frame 19 {
      n60 = for {
        tunnel: w750 -> [w762]
        tunnel: w736 -> [w752] mode=indexing
        tunnel: w749 -> [w754]
        tunnel: w748 -> [w756]
        tunnel: w747 -> [w768]
        tunnel: w746 -> [w767]
        tunnel: w745 -> [w766]
        tunnel: w744 -> [w765]
        tunnel: w743 -> [w764]
        tunnel: w742 -> [w763]
        tunnel: w741 -> [w760]
        tunnel: w740 -> [w759]
        tunnel: w739 -> [w758]
        tunnel: w738 -> [w757]
        tunnel: w735 -> [w755] mode=indexing
        tunnel: [w753] -> w737 mode=indexing
        tunnel: w734 -> [w751]
        i -> [w761]
        n61 = formula code="float ct;\n\nct=cdt*n+rmin;\n\nif (ct <= r3)\nh=cap[n]-asin(((z*loc[0]-x*loc[2])/(x**2+z**2)**0.5)/sig);\n\nelse if (ct < r1)\nh=2*cap[n];\n\nelse h=0;"("r0"=w768, "r1"=w767, "r2"=w766, "r3"=w765, "r4"=w764, "r5"=w763, "cdt"=w762, "n"=w761, "Pi"=w760, "x"=w759, "y"=w758, "z"=w757, "r"=w756, "sig"=w755, "loc"=w752, "cap"=w754, "rmin"=w751) -> ("h"=w753:dbl)
      }
    }
    frame 20 {
      n62 = for {
        tunnel: w785 -> [w797]
        tunnel: w771 -> [w787] mode=indexing
        tunnel: w784 -> [w789]
        tunnel: w783 -> [w791]
        tunnel: w782 -> [w803]
        tunnel: w781 -> [w802]
        tunnel: w780 -> [w801]
        tunnel: w779 -> [w800]
        tunnel: w778 -> [w799]
        tunnel: w777 -> [w798]
        tunnel: w776 -> [w795]
        tunnel: w775 -> [w794]
        tunnel: w774 -> [w793]
        tunnel: w773 -> [w792]
        tunnel: w770 -> [w790] mode=indexing
        tunnel: [w788] -> w772 mode=indexing
        tunnel: w769 -> [w786]
        i -> [w796]
        n63 = formula code="float ct;\n\nct=cdt*n+rmin;\n\nif (ct <= r3)\nh=acos((2*sig**2-(loc[0]**2+loc[1]**2+loc[2]**2))/(2*sig**2)+.000000003);\n\nelse if (ct < r4)\nh=cap[n]+asin(((z*loc[0]-x*loc[2])/(x**2+z**2)**0.5)/sig);\n\nelse if (ct < r1)\nh=2*cap[n];\n\nelse h=0;"("r0"=w803, "r1"=w802, "r2"=w801, "r3"=w800, "r4"=w799, "r5"=w798, "cdt"=w797, "n"=w796, "Pi"=w795, "x"=w794, "y"=w793, "z"=w792, "r"=w791, "sig"=w790, "loc"=w787, "cap"=w789, "rmin"=w786) -> ("h"=w788:dbl)
      }
    }
    frame 21 {
      n64 = for {
        tunnel: w820 -> [w832]
        tunnel: w806 -> [w822] mode=indexing
        tunnel: w819 -> [w824]
        tunnel: w818 -> [w826]
        tunnel: w817 -> [w838]
        tunnel: w816 -> [w837]
        tunnel: w815 -> [w836]
        tunnel: w814 -> [w835]
        tunnel: w813 -> [w834]
        tunnel: w812 -> [w833]
        tunnel: w811 -> [w830]
        tunnel: w810 -> [w829]
        tunnel: w809 -> [w828]
        tunnel: w808 -> [w827]
        tunnel: w805 -> [w825] mode=indexing
        tunnel: [w823] -> w807 mode=indexing
        tunnel: w804 -> [w821]
        i -> [w831]
        n65 = formula code="float ct;\n\nct=cdt*n+rmin;\n\nif (ct <= r4)\nh=2*cap[n];\n\nelse if (ct < r3)\nh=cap[n]-asin(((z*loc[0]-x*loc[2])/(x**2+z**2)**0.5)/sig);\n\n\nelse if (ct < r5)\nh=acos((2*sig**2-(loc[0]**2+loc[1]**2+loc[2]**2))/(2*sig**2)+.000000003);\n\nelse h=0;"("r0"=w838, "r1"=w837, "r2"=w836, "r3"=w835, "r4"=w834, "r5"=w833, "cdt"=w832, "n"=w831, "Pi"=w830, "x"=w829, "y"=w828, "z"=w827, "r"=w826, "sig"=w825, "loc"=w822, "cap"=w824, "rmin"=w821) -> ("h"=w823:dbl)
      }
    }
    frame 22 {
      # "case of x=0,y=0,z=0\n\nNeed to work with complex numbers.\n\nProbably don't need complex numbers but can leave them in."
      n66 = Sine(x=w857) -> (sin(x)=w858:dbl)
      n67 = formula code="b=2*a**2 - R**2 + R**2*cos(2*q);\nc=(2*a**2 - 2*R**2);\n\ng=-R*h*q;\nu=R**2;\np=R*sin(q)/a;\ne=R/2**.5;\n\n//compute 1/2 of area so need * 2\n\n f=2/(cdt*R**2);"("a"=w863, "R"=w865, "h"=w864, "q"=w857, "Pi"=w866, "cdt"=w846) -> ("f"=w848:dbl, "b"=w862:dbl, "c"=w861:dbl, "g"=w839:dbl, "e"=w853:dbl, "p"=w843:dbl, "u"=w841:dbl)
      n68 = To Double Precision Complex(1:w862) -> (0:w845:cdb)
      n69 = To Double Precision Complex(1:w861) -> (0:w851:cdb)
      n70 = To Double Precision Complex(1:w843) -> (0:w844:cdb)
      n71 = Square Root(x=w851) -> (sqrt(x)=w854:cdb)
      n72 = Square Root(x=w845) -> (sqrt(x)=w860:cdb)
      n73 = Divide(x=w854, y=w860) -> (x/y=w859:cdb)
      n74 = Inverse Sine(1:w844) -> (0:w842:cdb)
      n75 = Multiply(x=w858, y=w859) -> (x*y=w856:cdb)
      n76 = Multiply(x=w841, y=w842) -> (x*y=w840:cdb)
      n77 = Inverse Hyperbolic Tangent(1:w856) -> (0:w855:cdb)
      n78 = Compound Arithmetic op=MULTIPLY(w853, w854, w855) -> (w852:cdb)
      n79 = Compound Arithmetic op=ADD(w839, w840, w852) -> (w849:cdb)
      n80 = Multiply(x=w848, y=w849) -> (x*y=w850:cdb)
      n81 = Absolute Value(x=w850) -> (abs(x)=w847:dbl)
      n82 = Build Array(w847) -> (w867:dbl[])
    }
  }
  n83 = Equal?(x="Case Number", y=22) -> (x = y?=w12:bool)
  n84 = Select(t=1, s=w12, f=w8) -> (s? t:f=w11:dbl)
  n85 = Divide(x=w6, y=w11) -> (x/y=→"h wedge":dbl[])
  "slice delay out" <- "slice delay points in"
